vi "VS.UndeployError.Clear.vi"(8 "error in (no error)":errorcluster, 11 "WorkspaceManager in":T1) -> (0 "error out":errorcluster, 3 "WorkspaceManager  out":T1)   [LabVIEW 2015, in "Workspace.Obejct.Radio.lvlib"]
uses:
  Workspace.Obejct.Radio.lvlib
  <vilib>/NI Veristand/Execution/Workspace/WorkspaceAPI.ctl
  NationalInstruments.VeriStand.ClientAPI
  <vilib>/NI Veristand/Execution/Workspace/NI_VS Workspace ExecutionAPI.lvlib
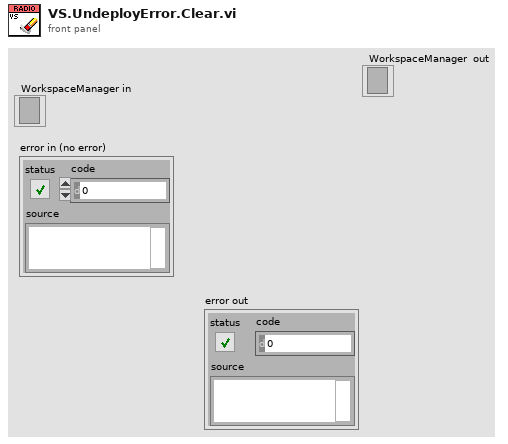
[diagram p1: front panel]
types:
  T1 = typedef "NI_VS Workspace ExecutionAPI.lvlib/WorkspaceAPI.ctl" = refnum<k24>
  T2 = typedef "NI_VS Workspace ExecutionAPI.lvlib/SystemState.ctl" = u8
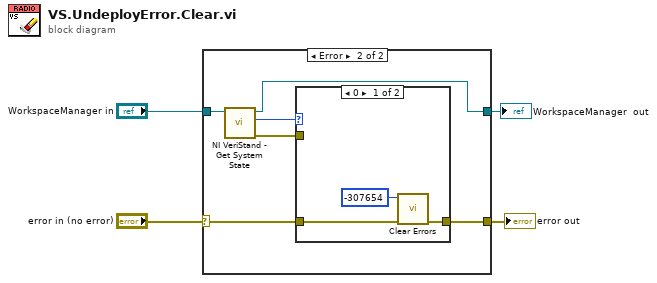
[diagram p0: block diagram]
diagram:
  n1 = case shown="Error" "error in (no error)" {
    selector: "error in (no error)" -> [w6 w8]
    tunnel: [w6 w11] -> w4
    tunnel: "WorkspaceManager in" -> [w5 w9]
    tunnel: [w5 w7] -> w1
    frame No Error {
    }
    frame Error {
      n2 = call <vilib>:"NI VeriStand - Get System State.vi"("WorkspaceManager in"=w9) -> ("error out"=w12:errorcluster, "System State"=w10:T2, "WorkspaceManager  out"=w7:T1)  [unwired: 6 in, 2 out]
      n3 = case shown="0" w10 {
        tunnel: [w15 w16] -> w11
        tunnel: w8 -> [w14 w16]
        tunnel: w12 -> [_ _]
        frame 0 {
          n4 = call <vilib>:"Clear Errors.vi"("error in (no error)"=w14, "specific error code to clear (0: all)"=-307654) -> ("error out"=w15:errorcluster)  [unwired: 4 in, 1 out]
        }
        frame Default {
        }
      }
    }
  }
  "error out" <- w4
  "WorkspaceManager  out" <- w1
